vi "JSONRPC-BuildError.vi"(9 "Message":string="Internal Error", 10 "Code":i32=-32603, 11 "ID":string) -> (3 "String":string)   [LabVIEW 2014]
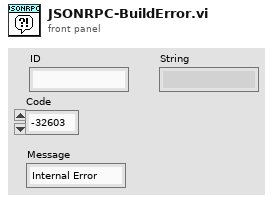
[diagram p1: front panel]
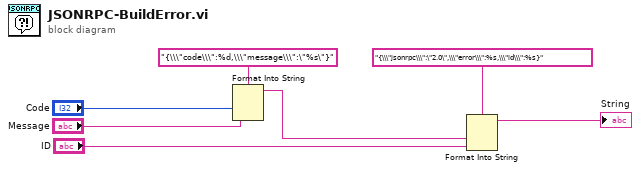
[diagram p0: block diagram]
diagram:
  n1 = Format Into String(format string="{\\\"code\\\":%d,\\\"message\\\":\"%s\"}", "Code", "Message") -> (resulting string=w5:string)  [unwired: 2 in, 1 out]
  n2 = Format Into String(format string="{\\\"jsonrpc\\\":\"2.0\",\\\"error\\\":%s,\\\"id\\\":%s}", w5, "ID") -> (resulting string=→"String":string)  [unwired: 2 in, 1 out]
